vi "IBM4_Write.vi"(8 "error in":errorcluster, 9 "Vset":dbl=1.0, 10 "Channel":i32, 11 "COM resource in":refnum<visa-resource-name>="COM9") -> (0 "error out":errorcluster, 3 "COM resource out":refnum<visa-resource-name>)   [LabVIEW 2021, in "IBM4.lvlib"]
doc: "Output a voltage (write) from the IBM4"
uses:
  <instrlib>/IBM4/IBM4.lvlib
  <vilib>/Instr/_visa.llb/VISA Configure Serial Port (Instr).vi
panel:
  out "read buffer":string
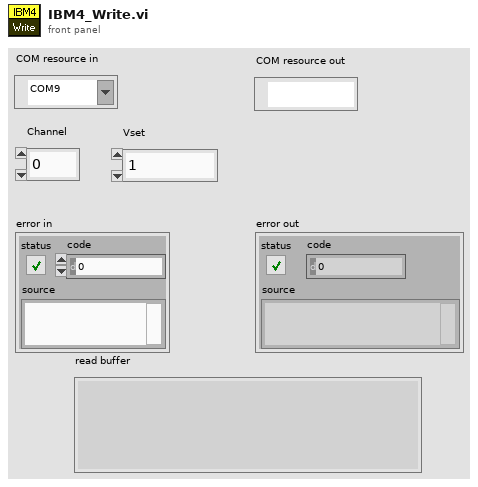
[diagram p1: front panel]
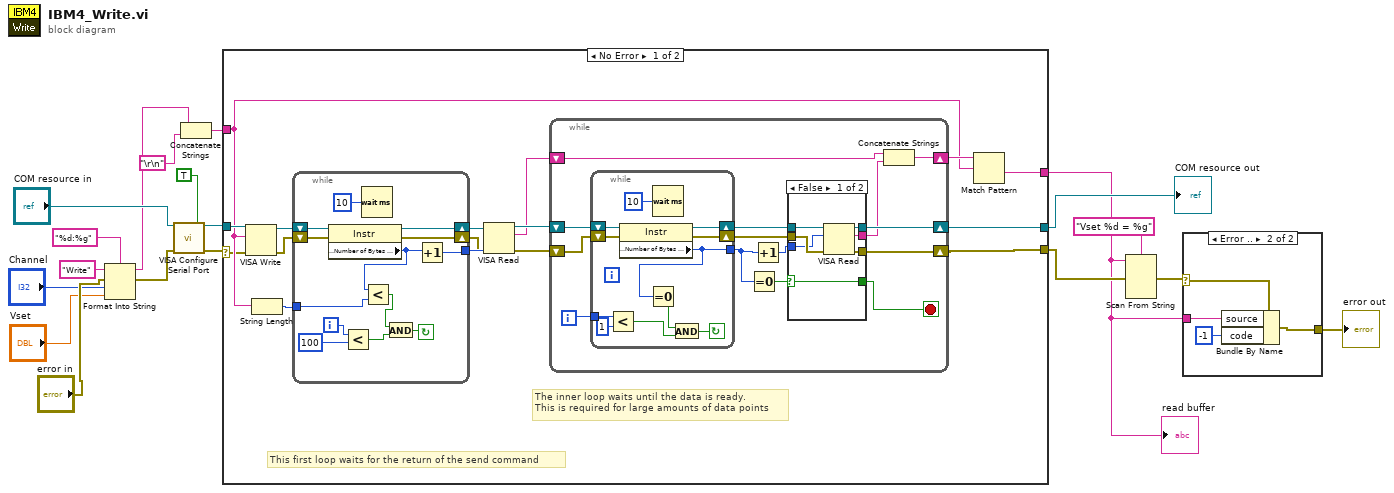
[diagram p0: block diagram]
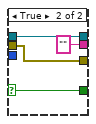
[diagram p3: hidden frame]
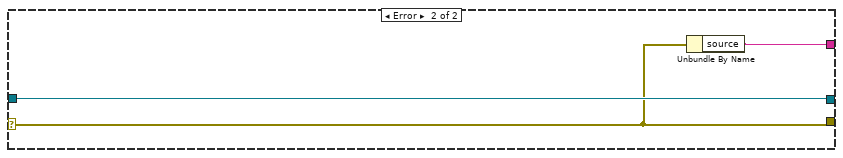
[diagram p4: hidden frame]
diagram:
  n1 = Format Into String(format string="%d:%g", initial string="Write", error in="error in", "Channel", "Vset") -> (resulting string=w5:string, error out=w14:errorcluster)
  n2 = call-poly "VISA Configure Serial Port"("VISA resource name"="COM resource in", "Enable Termination\nChar (T)"=TRUE ("Enable Termination\nChar (T)"), "error in (no error)"=w14) -> ("VISA resource name out"=w11:refnum<visa-resource-name>, "error out"=w10:errorcluster)  [unwired: 11 in]
  n3 = Concatenate Strings(w5, "\r\n") -> (w4:string)
  n4 = case shown="No Error" w10 {
    selector: w10 -> [w22 w85]
    tunnel: w11 -> [w35 w87]
    tunnel: [w21 w85] -> w8
    tunnel: [w33 w86] -> w1
    tunnel: w4 -> [w32 _]
    tunnel: [w20 w87] -> w9
    frame No Error {
      # "The inner loop waits until the data is ready.\nThis is required for large amounts of data points"
      # "This first loop waits for the return of the send command"
      n5 = VISA Write(VISA resource name=w35, write buffer=w32, error in (no error)=w22) -> (VISA resource name out=w31:refnum<visa-resource-name>, error out=w30:errorcluster)  [unwired: 1 out]
      n6 = String Length(string=w32) -> (length=w23:i32)
      n7 = while {
        tunnel: [w37] -> w28
        shift-right: [w47] -> w29
        shift-left: w31 -> [w48]
        shift-right: [w45] -> w27
        shift-left: w30 -> [w46]
        tunnel: w23 -> [w43]
        i -> [w38]
        stop <- w41 continue-if-true
        n8 = property class="Instr"(reference=w48, error in=w46) -> (reference out=w47:refnum<visa-resource-name>, error out=w45:errorcluster, "Serial Settings:Number of Bytes at Serial Port"=w36:u32)
        n9 = Less?(x=w38, y=100) -> (x < y?=w40:bool)
        n10 = Wait (ms)(milliseconds to wait=u32 10) -> ()  [unwired: 1 out]
        n11 = Less?(x=w36, y=w43) -> (x < y?=w39:bool)
        n12 = And(x=w39, y=w40) -> (x .and. y?=w41:bool)
        n13 = Increment(x=w36) -> (x+1=w37:u32)
      }
      n14 = VISA Read(VISA resource name=w29, byte count=w28, error in (no error)=w27) -> (VISA resource name out=w26:refnum<visa-resource-name>, read buffer=w24:string, error out=w25:errorcluster)  [unwired: 1 out]
      n15 = while {
        shift-right: [w62] -> w20
        shift-left: w26 -> [w60]
        shift-right: [w61] -> w21
        shift-left: w25 -> [w58]
        shift-right: [w56] -> w34
        shift-left: w24 -> [w54]
        i -> [w53]
        stop <- w49 stop-if-true
        n16 = while {
          tunnel: [w79] -> w52
          shift-right: [w83] -> w59
          shift-left: w60 -> [w84]
          shift-right: [w81] -> w57
          shift-left: w58 -> [w82]
          tunnel: w53 -> [w78]
          stop <- w76 continue-if-true
          n17 = Less?(x=w78, y=1) -> (x < y?=w75:bool)
          n18 = property class="Instr"(reference=w84, error in=w82) -> (reference out=w83:refnum<visa-resource-name>, error out=w81:errorcluster, "Serial Settings:Number of Bytes at Serial Port"=w79:u32)
          n19 = Equal To 0?(x=w79) -> (x = 0?=w74:bool)
          n20 = Wait (ms)(milliseconds to wait=u32 10) -> ()  [unwired: 1 out]
          n21 = And(x=w74, y=w75) -> (x .and. y?=w76:bool)
        }
        n22 = Equal To 0?(x=w52) -> (x = 0?=w50:bool)
        n23 = Increment(x=w52) -> (x+1=w51:u32)
        n24 = case shown="False" w50 {
          selector: w50 -> [w63 w72]
          tunnel: [w69 w73] -> w62
          tunnel: [w68 w71] -> w61
          tunnel: w59 -> [w67 w73]
          tunnel: w57 -> [w66 w71]
          tunnel: [w65 "" ("read buffer")] -> w55
          tunnel: w51 -> [w64 _]
          tunnel: [w63 w72] -> w49
          frame False {
            n25 = VISA Read(VISA resource name=w67, byte count=w64, error in (no error)=w66) -> (VISA resource name out=w69:refnum<visa-resource-name>, read buffer=w65:string, error out=w68:errorcluster)  [unwired: 1 out]
          }
          frame True {
          }
        }
        n26 = Concatenate Strings(w54, w55) -> (w56:string)
      }
      n27 = Match Pattern(string=w34, regular expression=w32) -> (after substring=w33:string)  [unwired: 1 in, 3 out]
    }
    frame Error {
      n28 = Unbundle By Name(w85) -> ("source"=w86:string)
    }
  }
  "COM resource out" <- w9
  "read buffer" <- w1
  n29 = Scan From String(format string="Vset %d = %g", input string=w1, error in=w8) -> (error out=w3:errorcluster)  [unwired: 5 in, 2 out]
  n30 = case shown="Error .." w3 {
    selector: w3 -> [w88 w92]
    tunnel: [w88 w90] -> w2
    tunnel: w1 -> [_ w91]
    frame No Error {
    }
    frame Error {
      n31 = Bundle By Name(cluster=w92, "source"=w91, "code"=-1) -> (w90:errorcluster)
    }
  }
  "error out" <- w2
